vi "Decode payload.vi"(8 "error in (no error)":errorcluster, 11 "JSONWebToken in":refnum<class "JSONWebToken.lvclass">) -> (0 "error out":errorcluster, 2 "JTW Claims (JSON)":string, 3 "JSONWebToken out":refnum<class "JSONWebToken.lvclass">)   [LabVIEW 2024]
uses:
  JSONWebToken.lvclass/JSONWebToken.ctl
  <vilib>/JDP Science/JSONtext/JSONtext.lvlib
  JSONWebToken.lvclass
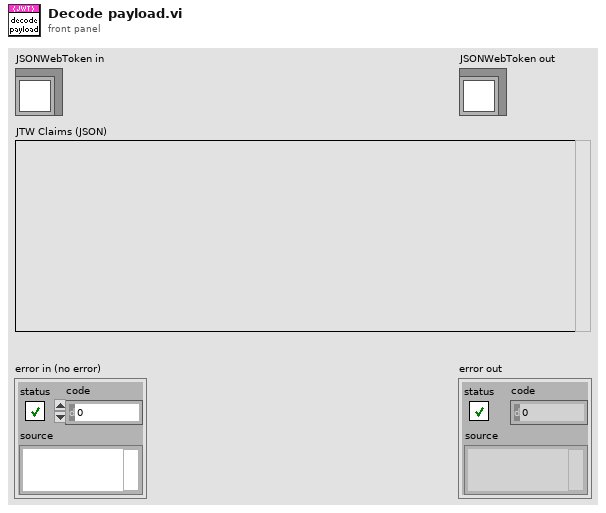
[diagram p1: front panel]
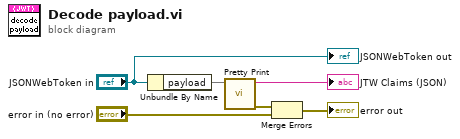
[diagram p0: block diagram]
diagram:
  n1 = Unbundle By Name("JSONWebToken in") -> ("payload"=w3)
  n2 = call <vilib>:"Pretty Print.vi"("JSON"=w3) -> ("error out"=w6:errorcluster, "<JSON>"=→"JTW Claims (JSON)":string)  [unwired: 8 in, 1 out]
  n3 = Merge Errors(w6, "error in (no error)") -> (→"error out":errorcluster)
  "JSONWebToken out" <- "JSONWebToken in"
